vi "weighPlatforms.vi"(11 "platforms":i32[](array[numeric])) -> (3 "weights":dbl[](array[numeric]))   [LabVIEW 2017]
panel:
  out "Separated inputs\nas strings":string[](array[string])
  out "voltsPerGram":dbl[](array[numeric])
  out "zeroSignals":dbl[](array[numeric])
  out "load cell\nsignal":dbl[](array[numeric])
  # "Channels to weigh"
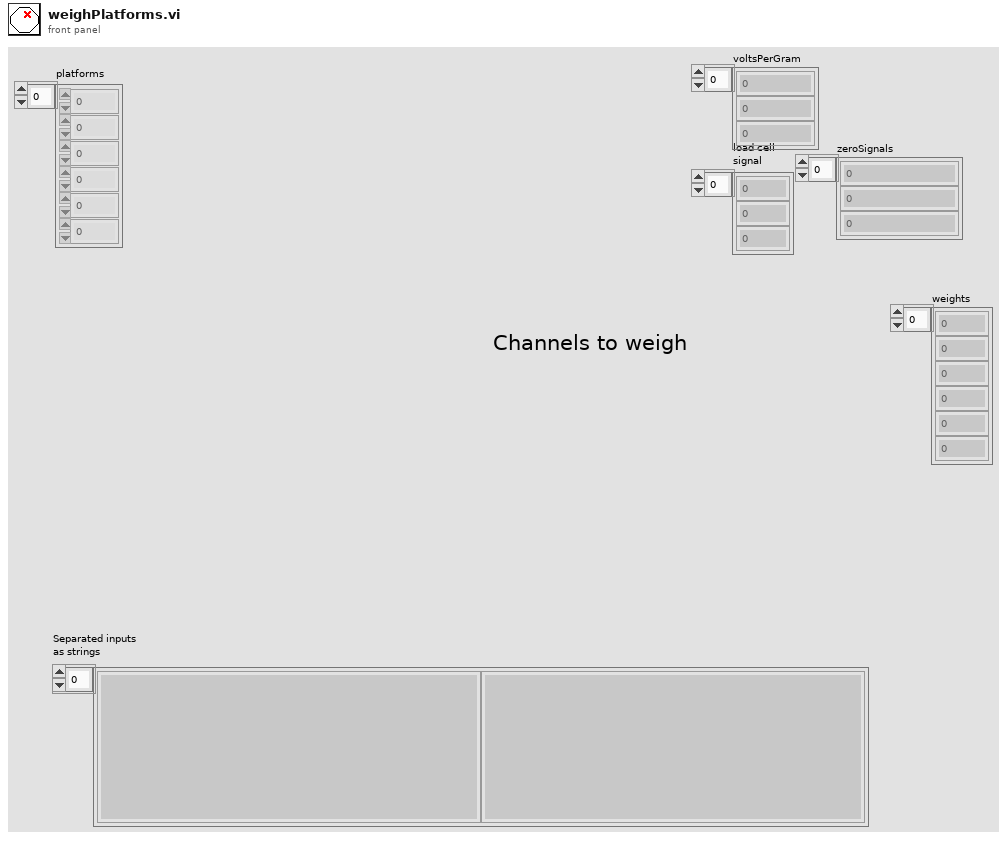
[diagram p1: front panel]
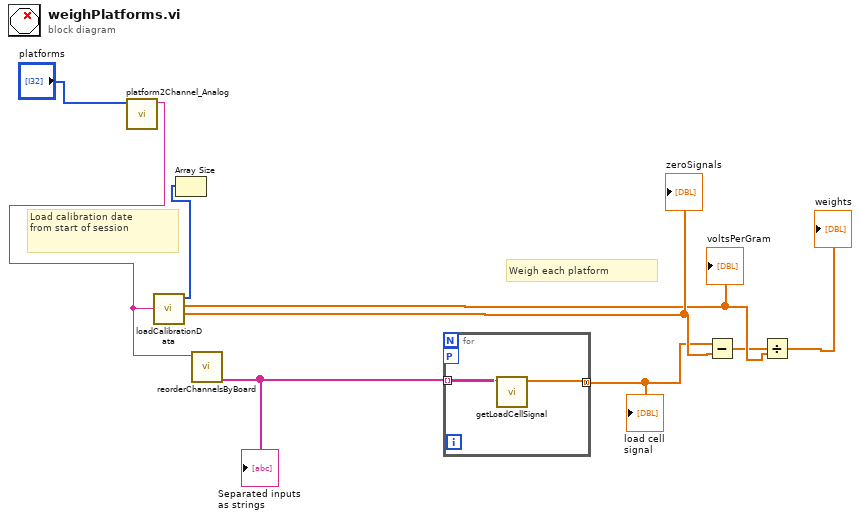
[diagram p0: block diagram]
diagram:
  # "Weigh each platform"
  # "Load calibration date\nfrom start of session"
  n1 = call "platform2Channel_Analog.vi"("platforms"="platforms") -> ("DAQmx Channel"=w4:string)  [unwired: 10 in]
  n2 = call "loadCalibrationData.vi"("DAQmx \nPhysical Channel"=w4) -> ("zeroSignals"=w9:dbl[], "voltsPerGram"=w8:dbl[], "index"=w6:i32[])  [unwired: 7 in, 1 out]
  "zeroSignals" <- w9
  "voltsPerGram" <- w8
  n3 = Array Size(array=w6) -> ()  [unwired: 1 out]
  n4 = call "reorderChannelsByBoard.vi"("DAQmx \nPhysical Channel"=w4) -> ("Separated inputs\nas strings"=w7:string[])  [unwired: 8 in, 2 out]
  "Separated inputs\nas strings" <- w7
  n5 = for {
    workers-P: _ -> [_]
    tunnel: w7 -> [w11] mode=indexing
    tunnel: [w10] -> w2 mode=concatenating
    n6 = call "getLoadCellSignal.vi"("DAQmx Physical Channel"=w11) -> ("load cell\nsignal"=w10:dbl[])  [unwired: 10 in]
  }
  "load cell\nsignal" <- w2
  n7 = Subtract(x=w2, y=w9) -> (x-y=w3:dbl[])
  n8 = Divide(x=w3, y=w8) -> (x/y=→"weights":dbl[])
